vi "While Loop Sine Wave Graph.vi"() -> ()   [LabVIEW 2017]
panel:
  out "Array":dbl[](array[numeric])
  out "Waveform Graph":cluster{dbl, dbl, dbl[]}(graph)
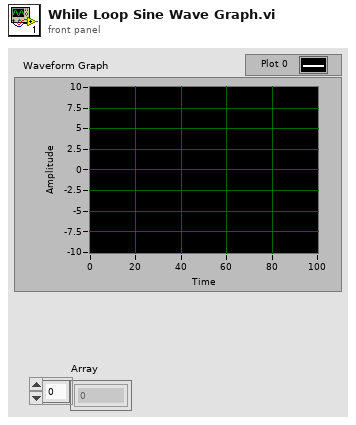
[diagram p1: front panel]
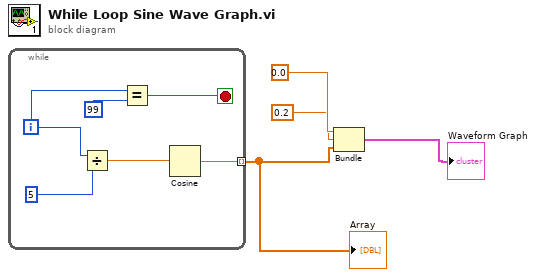
[diagram p0: block diagram]
diagram:
  n1 = while {
    tunnel: [w5] -> w1 mode=indexing
    i -> [w9]
    stop <- w7 stop-if-true
    n2 = Divide(x=w9, y=5) -> (x/y=w6:dbl)
    n3 = Equal?(x=w9, y=99) -> (x = y?=w7:bool)
    n4 = Cosine(x=w6) -> (cos(x)=w5:dbl)
  }
  "Array" <- w1
  n5 = Bundle(0.0, 0.2, w1) -> (→"Waveform Graph":cluster{dbl, dbl, dbl[]})  [unwired: 1 in]
